vi "zad1.vi"() -> ()   [LabVIEW 2017]
panel:
  out "Numeric 2":dbl
  out "Numeric":dbl
  in  "OK Button":bool
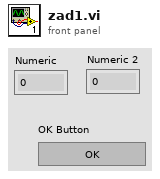
[diagram p1: front panel]
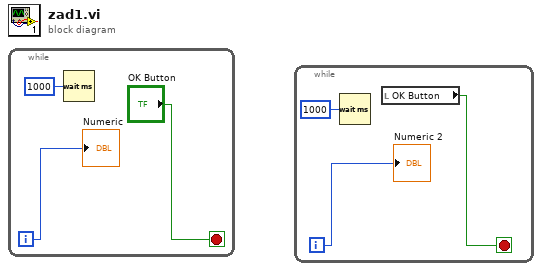
[diagram p0: block diagram]
diagram:
  n1 = while {
    i -> [w3]
    stop <- "OK Button" stop-if-true
    n2 = Wait (ms)(milliseconds to wait=u32 1000) -> ()  [unwired: 1 out]
    "Numeric" <- w3
  }
  n3 = while {
    i -> [w6]
    stop <- w5 stop-if-true
    n4 = Wait (ms)(milliseconds to wait=u32 1000) -> ()  [unwired: 1 out]
    n5 = local read "OK Button"() -> (w5:bool)
    "Numeric 2" <- w6
  }
